vi "csuShutterState.vi"() -> (6 "Open":bool)   [LabVIEW 2017]
doc: "SubVI for sending commands to the MAC5000 and receiving responses from the MAC5000."
uses:
  globalDevices.vi
panel:
  out "Raw Response":string
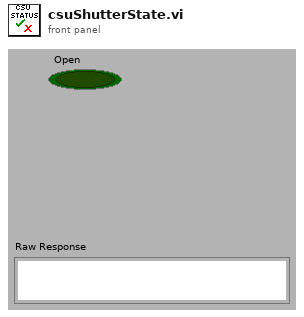
[diagram p1: front panel]
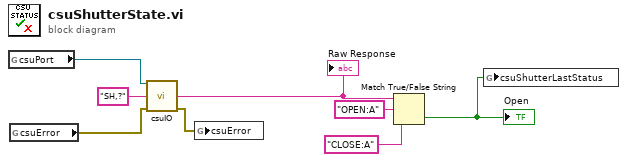
[diagram p0: block diagram]
diagram:
  n1 = global read "globalDevices.vi" "csuPort"() -> (w4:refnum<visa-resource-name>)
  n2 = global read "globalDevices.vi" "csuError"() -> (w3:errorcluster)
  n3 = call "csuIO.vi"("VISA  IN"=w4, "Command (to ctlr)"="SH,?", "error in"=w3) -> ("Raw Response"=w7:string, "error out"=w2:errorcluster)  [unwired: 9 in, 2 out]
  "Raw Response" <- w7
  n4 = global write "globalDevices.vi" "csuError"(w2) -> ()
  n5 = Match True/False String(2:"CLOSE:A" ("false string"), 3:"OPEN:A" ("true string"), 4:w7) -> (0:w1:bool)  [unwired: 1 out]
  "Open" <- w1
  n6 = global write "globalDevices.vi" "csuShutterLastStatus"(w1) -> ()
